vi "Get Config File Path.vi"(8 "error in":errorcluster) -> (0 "error out":errorcluster, 3 "XML File Path":path)   [LabVIEW 2020, in "Settings Editor.lvlib"]
doc: "Get the path to the Settings XML file. This is done using the Application Directory function. For more information on how Application Directory calculates its path, right-click the function and choose Help.\n_____\nBased on DQMH Project Template 7.0.1.1316."
uses:
  Settings Editor.lvlib
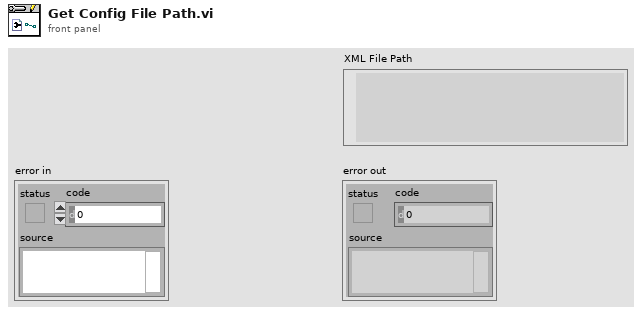
[diagram p1: front panel]
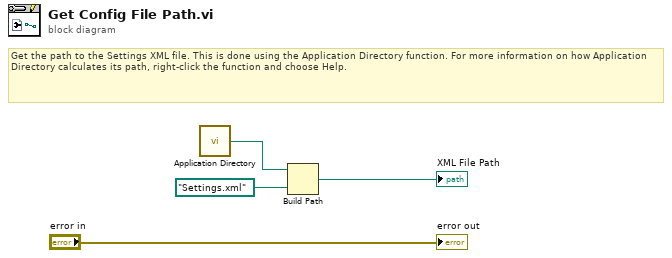
[diagram p0: block diagram]
diagram:
  # "Get the path to the Settings XML file. This is done using the Application Directory function. For more information on how Application Directory calculates its path, right-click the function and choose Help."
  n1 = call <vilib>:"Application Directory.vi"() -> ("Application Directory"=w1:path)
  n2 = Build Path(base path=w1, name or relative path=path "Settings.xml" ("string")) -> (appended path=→"XML File Path":path)
  "error out" <- "error in"
